vi "Send data by Email.vi"(3 "to":string="yehtingo@gmail.com", 4 "Attachment?":bool, 5 "plain text message":string="works?", 6 "Attachment path":path, 7 "subject":string="Test", 8 "error in":errorcluster, 9 "APP password":string="aiwfjsidudnfefes\n", 10 "username":string="ncuccc45002931", 11 "from":string="ncuccc45002931@gmail.com") -> (0 "error out":errorcluster)   [LabVIEW 2023]
uses:
  <vilib>/smtpClient/Set Message Text.vi
  <vilib>/smtpClient/LabVIEWSMTPClient.lvlib
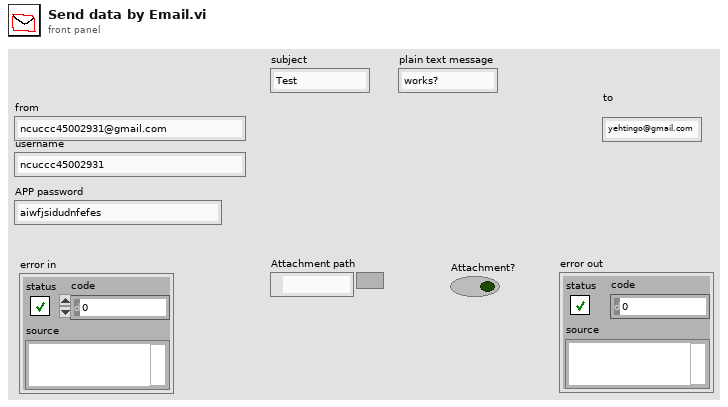
[diagram p1: front panel]
types:
  T1 = typedef "LabVIEWSMTPClient.lvlib/SmtpClientHandle.ctl" = refnum<k1>
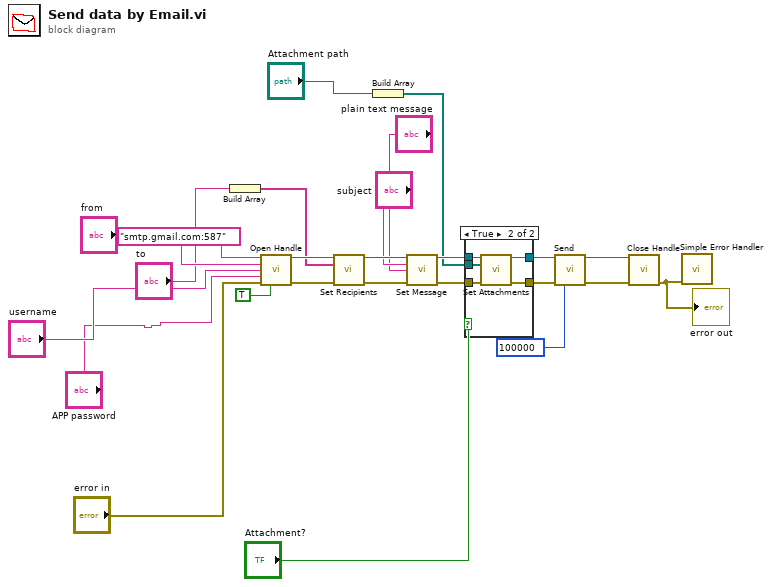
[diagram p0: block diagram]
diagram:
  n1 = Build Array("to") -> (w11:string[])
  n2 = call <vilib>:"Open Handle.vi"("server address"="smtp.gmail.com:587", "from"="from", "username"="username", "password"="APP password", "error in (no error)"="error in", "use TLS (false)"=TRUE) -> ("handle out"=w25:T1, "error out"=w24:errorcluster)  [unwired: 8 in]
  n3 = call <vilib>:"Set Recipients.vi"("handle in"=w25, "to"=w11, "error in (no error)"=w24) -> ("handle out"=w23:T1, "error out"=w22:errorcluster)  [unwired: 11 in]
  n4 = Build Array("Attachment path") -> (w6:path[])
  n5 = call-poly <vilib>:"Set Message.vi"("handle in"=w23, "subject"="subject", "plain text message"="plain text message", "error in (no error)"=w22) -> ("handle out"=w21:T1, "error out"=w20:errorcluster)  [unwired: 10 in]
  n6 = case shown="True" "Attachment?" {
    tunnel: w21 -> [w27 w32]
    tunnel: w20 -> [w26 w31]
    tunnel: [w27 w30] -> w19
    tunnel: [w26 w29] -> w18
    tunnel: w6 -> [_ w28]
    frame False {
    }
    frame True {
      n7 = call <vilib>:"Set Attachments.vi"("handle in"=w32, "attachments"=w28, "error in (no error)"=w31) -> ("handle out"=w30:T1, "error out"=w29:errorcluster)  [unwired: 11 in]
    }
  }
  n8 = call <vilib>:"Send.vi"("handle in"=w19, "error in (no error)"=w18, "timeout in ms (10000)"=100000) -> ("handle out"=w17:T1, "error out"=w16:errorcluster)  [unwired: 10 in, 1 out]
  n9 = call <vilib>:"Close Handle.vi"("handle in"=w17, "error in (no error)"=w16) -> ("error out"=w15:errorcluster)  [unwired: 12 in, 1 out]
  "error out" <- w15
  n10 = call <vilib>:"Simple Error Handler.vi"("error in (no error)"=w15) -> ()  [unwired: 4 in, 5 out]
